vi "set_sp_data.vi"(0 "yw":string, 4 "sp_shuoming":string, 6 "sp_yijian":string, 8 "sp_ren":string, 9 "cur_spsta":string, 10 "lc_num":string, 11 "pro_spnum":string) -> (1 "error":errorcluster caption="error out 2", 2 "spnum":string)   [LabVIEW 2017, in "Lib_code.lvlib"]
uses:
  Lib_code.lvlib
panel:
  out "error":errorcluster caption="error out 2"
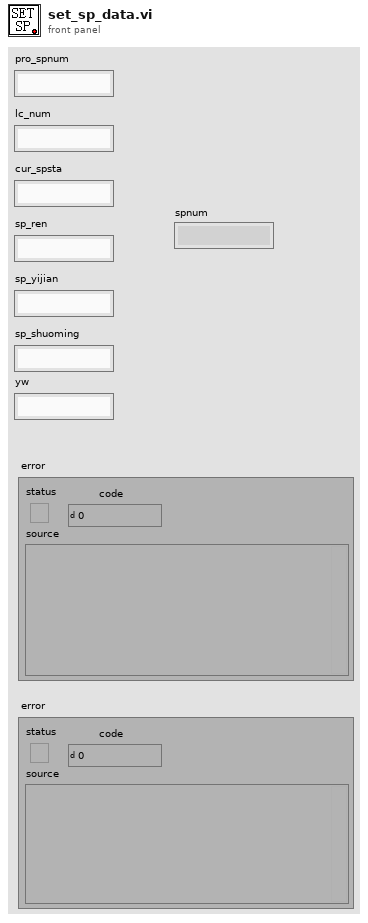
[diagram p1: front panel]
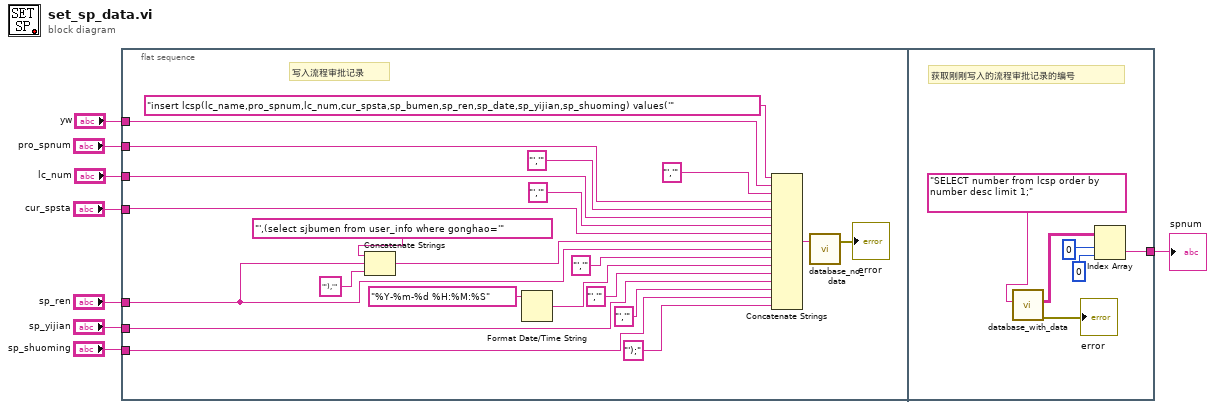
[diagram p0: block diagram]
diagram:
  n1 = flat-sequence {
    tunnel: "lc_num" -> [w25]
    tunnel: "sp_yijian" -> [w9]
    tunnel: "sp_shuoming" -> [w23]
    tunnel: "sp_ren" -> [w17]
    tunnel: "cur_spsta" -> [w16]
    tunnel: "pro_spnum" -> [w15]
    tunnel: "yw" -> [w11]
    tunnel: [w34] -> w5
    frame #0 {
      # "写入流程审批记录"
      n2 = Concatenate Strings("',(select sjbumen from user_info where gonghao='" ("Command Text"), w17, "'),'" ("字符串")) -> (w18:string)
      n3 = Format Date/Time String(time format string (%c)="%Y-%m-%d %H:%M:%S" ("时间格式字符串(%c)")) -> (date/time string=w21:string)  [unwired: 2 in]
      n4 = Concatenate Strings("insert lcsp(lc_name,pro_spnum,lc_num,cur_spsta,sp_bumen,sp_ren,sp_date,sp_yijian,sp_shuoming) values('" ("格式字符串"), w11, "','" ("字符串"), w15, "','" ("字符串"), w25, "','" ("字符串"), w16, w18, w17, "','" ("字符串"), w21, "','" ("字符串"), w9, "','" ("字符串"), w23, "');" ("字符串")) -> (w13:string)
      n5 = call "database_no_data.vi"("input"=w13) -> ("error"=→"error":errorcluster)  [unwired: 2 in]
    }
    frame #1 {
      # "获取刚刚写入的流程审批记录的编号"
      n6 = call "database_with_data.vi"("input"="SELECT number from lcsp order by number desc limit 1;" ("Command Text")) -> ("error"=→"error":errorcluster, "Data"=w33:string[][])  [unwired: 9 in]
      n7 = Index Array(array=w33, index (row)=0 ("索引 (行)"), index (col)=0 ("禁用的索引 (列)")) -> (element=w34:string)
    }
  }
  "spnum" <- w5
